vi "RDB Create Objects Sent.vi"(8 "error in (no error)":errorcluster, 11 "RDB Data Sent":T1) -> (0 "error out":errorcluster, 3 "RDB Send Reference":refnum<class "DataContainer.lvclass">)   [LabVIEW 2023, in "RDB.lvlib"]
uses:
  RDB.lvlib
  System Explorer/RDB Data.ctl
  RDB Object.ctl
  RDB Player Object.ctl
  DataContainer/DataContainer.lvclass
  <vilib>/xnet/xnet.llb/XNET Frame FlexRay.ctl
  <vilib>/xnet/xnet.llb/XNET Frame Type FlexRay.ctl
  <vilib>/xnet/xnet.llb/XNET String To IO Name (Signal).vi
  <vilib>/xnet/xnet.llb/XNET Create Session (Conversion).vi
  <resource>/objmgr/xnet.rc
  Shared/Vires VTD Shared.lvlib
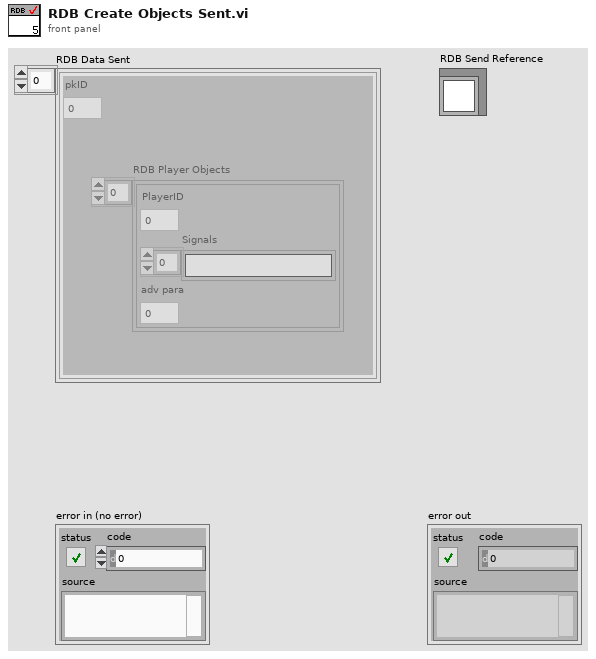
[diagram p1: front panel]
types:
  T1 = typedef "Vires VTD Shared.lvlib/RDB Data.ctl" = T2[]
  T2 = typedef "RDB.lvlib/RDB Object.ctl" = cluster{"pkID":i32, "RDB Player Objects":T3[]}
  T3 = typedef "RDB.lvlib/RDB Player Object.ctl" = cluster{"PlayerID":i32, "Signals":string[], "adv para":i32}
  T4 = typedef "XNET Frame FlexRay.ctl" = cluster{"timestamp":timestamp, "payload":u8[], "slot":u16, "type":T5, "cycle count":u8, "startup?":bool, "sync?":bool, "preamble?":bool, "ch A":bool, "ch B":bool, "echo?":bool}
  T5 = typedef "XNET Frame Type FlexRay.ctl" = u8
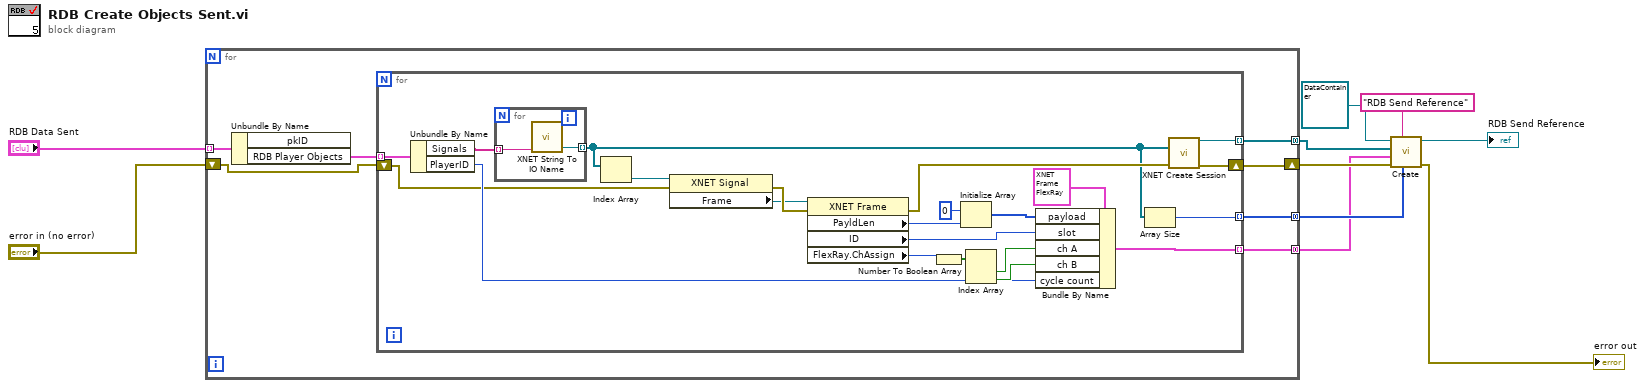
[diagram p0: block diagram]
diagram:
  n1 = for {
    tunnel: "RDB Data Sent" -> [w17] mode=indexing
    shift-right: [w15] -> w4
    shift-left: "error in (no error)" -> [w14]
    tunnel: [w13] -> w7 mode=concatenating
    tunnel: [w12] -> w2 mode=concatenating
    tunnel: [w11] -> w8 mode=concatenating
    n2 = Unbundle By Name(w17) -> ("RDB Player Objects"=w16:T3[])  [unwired: 1 out]
    n3 = for {
      tunnel: w16 -> [w39] mode=indexing
      tunnel: [w24] -> w12 mode=indexing
      tunnel: [w20] -> w13 mode=indexing
      shift-right: [w22] -> w15
      shift-left: w14 -> [w21]
      tunnel: [w18] -> w11 mode=indexing
      n4 = Unbundle By Name(w39) -> ("Signals"=w38:string[], "PlayerID"=w25:i32)
      n5 = for {
        tunnel: w38 -> [w41] mode=indexing
        tunnel: [w40] -> w19 mode=indexing
        n6 = call-poly <vilib>:"XNET String To IO Name.vi"("string"=w41) -> ("XNET Signal"=w40:refnum<k21>)  [unwired: 4 out]
      }
      n7 = Index Array(array=w19) -> (element=w26:refnum<k21>)  [unwired: 1 in]
      n8 = property class="XNET Signal"(reference=w26, error in=w21) -> (error out=w37:errorcluster, "Frame"=w36:refnum<k21>)  [unwired: 1 out]
      n9 = property class="XNET Frame"(reference=w36, error in=w37) -> (error out=w23:errorcluster, "PayldLen"=w29:u32, "ID"=w31:u32, "FlexRay.ChAssign"=w32:u32)  [unwired: 1 out]
      n10 = Number To Boolean Array(number=w32) -> (Boolean array=w27:bool[])
      n11 = Initialize Array(u8 0 ("element"), w29) -> (w30:u8[])
      n12 = Index Array(array=w27) -> (element #1=w33:bool, element #2=w34:bool)  [unwired: 2 in]
      n13 = Bundle By Name(cluster=T4 {"timestamp"=timestamp(0 s since 1904-01-01), "payload"=[], "slot"=1, "type"=32, "cycle count"=0, "startup?"=FALSE, "sync?"=FALSE, "preamble?"=FALSE, "ch A"=FALSE, "ch B"=FALSE, "echo?"=FALSE} ("FlexRay frame"), "payload"=w30, "slot"=w31, "ch A"=w33, "ch B"=w34, "cycle count"=w25) -> (w24:T4)
      n14 = Array Size(array=w19) -> (size(s)=w18:i32)
      n15 = call-poly <vilib>:"XNET Create Session.vi"("signal list"=w19, "error in (no error)"=w23) -> ("session out"=w20:refnum<k21>, "error out"=w22:errorcluster)  [unwired: 12 in]
    }
  }
  n16 = call-dynamic "Create.vi"("noSignals"=w8, "Container ID"="RDB Send Reference", "error in (no error)"=w4, "Package Data"=w2, "Conversion References"=w7, "DataContainer in"=refnum<class "DataContainer.lvclass"> refnum) -> ("error out"=→"error out":errorcluster, "DataContainer out"=→"RDB Send Reference":refnum<class "DataContainer.lvclass">)  [unwired: 4 in]
